vi "OAT Spectral Map (2D array).vi"(0 "scaled signal [EU]":waveform(dbl)={"t0"=timestamp(0 s since 1904-01-01), "dt"=0.0, "Y"=[]}, 1 "dB on? (T)":bool=TRUE, 2 "reset? (F)":bool, 3 "plot type":T9(ring), 5 "speed profile":T8 {"speed [RPM]" format="%.2f"; "time [s]" format="%.2f"}, 7 "pulse/revolution (1)":i32=1, 9 "time/speed segment [s or RPM]":cluster{"start":dbl, "end":dbl, "step size":dbl} {"step size" format="%.2f"; "end" min=0.0 format="%.2f"; "start" min=0.0 format="%.2f"}, 11 "error in (no error)":errorcluster, 12 "max order (auto)":dbl, 13 "windows info":cluster{"window type":u32, "window length":i32}={"window type"=62, "window length"=2048} {"window length" min=2; "window type" items=["None"=0, "Hanning"=1, "Hamming"=2, "Blackman-Harris"=3, "Exact Blackman"=4, "Blackman"=5, "Flat Top"=6, "4 Term B-Harris"=7, "7 Term B-Harris"=8, "Low Sidelobe"=9, "Gaussian"=62]}) -> (4 "spectral map":dbl[][](array[numeric]) format="%.2f", 6 "spectral map info":T7={"scales"={"x scale"={"offset"=0.0, "multiplier"=0.0}, "y scale"={"offset"=0.0, "multiplier"=0.0}}, "unit labels"={"x-axis unit label"="", "y-axis unit label"="", "z-axis unit label"=""}, "plot type"=enum."Frequency-Time", "dB on"=TRUE} {"scales"."y scale"."multiplier" format="%.2f"; "scales"."y scale"."offset" format="%.2f"; "scales"."x scale"."multiplier" format="%.2f"; "scales"."x scale"."offset" format="%.2f"}, 8 "spectrum info":T1={"channel name"="", "description"="", "x-axis units"=0, "spectral info"={"spectrum type"=enum."Power [Magnitude^2]", "linear/dB"=enum."linear", "window"=0, "window size"=0, "FFT size"=0}, "engineering units"=0, "custom label"="", "dB reference [EU]"=0.0, "peak units"=enum."rms", "weighting filter"=0, "spectral density?"=FALSE, "unit label"="", "spectrum skewed?"=FALSE, "complimentary spectrum units"=enum."none"} {"x-axis units" items=["Time (s)"=0, "Frequency-CB (Hz)"=1, "Frequency-CPB (Hz)"=1248, "Frequency-Arbitrary (Hz)"=2357, "Quefrency (s)"=2, "Revolutions (rev)"=3, "Order"=4, "Speed (RPM)"=11, "Speed (rad/s)"=21, "Index"=65535]; "weighting filter" items=["Linear", "A-weighting", "B-weighting", "C-weighting", "ITU-R 468-4", "Dolby", "CCITT", "C-message", "Wb", "Wc", "Wd", "We", "Wf", "Wh", "Wj", "Wk", "Wm", "AES17 20 kHz lowpass", "AES17 40 kHz lowpass", "AES17 20 kHz highpass", "AES17 40 kHz highpass"]; "dB reference [EU]" format="%.2f"; "engineering units" items=["custom..."=0, "V"=1, "A"=21, "C"=30, "pC"=31, "s"=32, "-"=29, "Pa"=2, "N"=20, "g"=3, "m/s^2"=4, "m/s"=5, "m"=6, "mm/s"=12, "mm"=13, "micron/s"=14, "micron"=15, "in/s^2"=7, "in/s"=8, "in"=9, "mil/s"=10, "mil"=11, "rad/s^2"=16, "rad/s"=17, "rad"=18, "deg/s^2"=26, "deg/s"=27, "deg"=28, "RPM"=22, "cycle/s^2"=23, "Hz"=24, "cycle"=25, "strain"=19]; "spectral info"."window" items=["None "=0, "Hanning"=1, "Hamming"=2, "Blackman-Harris"=3, "Exact Blackman"=4, "Blackman"=5, "Flat Top"=6, "4 Term B-Harris "=7, "7 Term B-Harris"=8, "Low Sidelobe"=9, "Force - Exponential"=10, "Gaussian"=62]}, 10 "end reached?":bool, 15 "error out":errorcluster)   [LabVIEW 2017, in "SoundVib_OrderTracking.lvlib"]
doc: "Computes a spectral map of the <B>scaled signal [EU]</B> as a function of time or rotational speed. This VI can return the spectral map as a 2D numeric array, a colormap, or a waterfall graph. Wire data to the <B>scaled signal [EU]</B> input to determine the polymorphic instance to use or manually select the instance."
uses:
  <vilib>/addons/Sound and Vibration/Order Analysis/Resample Order Tracking/SoundVib_OrderTracking.lvlib
  <vilib>/addons/Sound and Vibration/Order Analysis/Tach Process/SubVIs/speed profile.ctl
  <vilib>/addons/Sound and Vibration/Order Analysis/Resample Order Tracking/SubVIs/Spectral Map Info.ctl
  <vilib>/addons/_NISVFA/_Shared subVIs/Controls/svc_Spectrum Info.ctl
  <vilib>/addons/_NISVFA/_Shared subVIs/Controls/svc_X-Axis Units.ctl
  <vilib>/addons/_NISVFA/_Shared subVIs/Controls/svc_Spectrum Type.ctl
  <vilib>/addons/_NISVFA/_Shared subVIs/Controls/svc_Engineering Units Text Ring.ctl
  <vilib>/addons/_NISVFA/_Shared subVIs/Controls/svc_Weighting Filter Text Ring.ctl
  <vilib>/addons/_NISVFA/_Shared subVIs/Controls/svc_Complimentary Spectrum Units.ctl
  <vilib>/addons/_NISVFA/_Shared subVIs/Common/svc_Check for Waveform Parameter Continuity (no state).vi
  <vilib>/addons/Sound and Vibration/Order Analysis/Resample Order Tracking/OAT Convert to Even Angle Signal (1 Channel).vi
  <vilib>/addons/_NISVFA/_Shared subVIs/Common/svc_Engineering Units to Unit Label.vi
  <vilib>/addons/_NISVFA/_Shared subVIs/Common/svc_Unit Label to Engineering Units.vi
  <vilib>/addons/Sound and Vibration/Order Analysis/Resample Order Tracking/SoundVib_Resampling.lvlib
  <vilib>/addons/Sound and Vibration/Order Analysis/Tach Process/SoundVib_TachProcess.lvlib
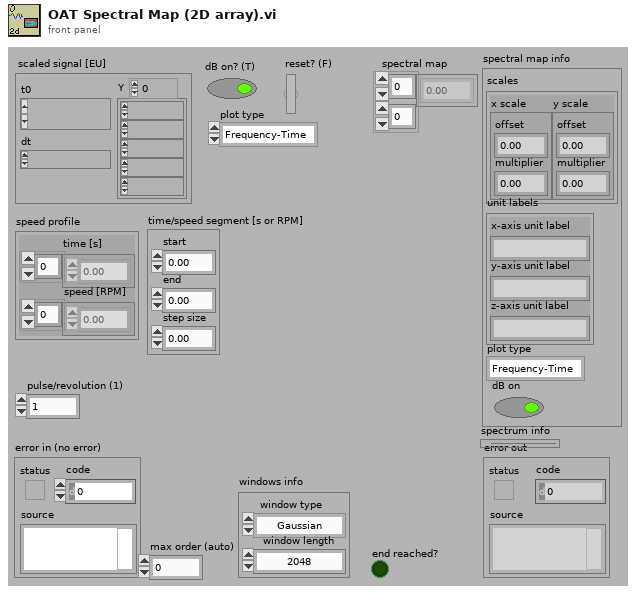
[diagram p1: front panel]
types:
  T1 = typedef "svc_Spectrum Info.ctl" = cluster{"channel name":string, "description":string, "x-axis units":T2, "spectral info":cluster{"spectrum type":T3, "linear/dB":enum16{"linear", "dB"}, "window":u16, "window size":i32, "FFT size":i32}, "engineering units":T4, "custom label":string, "dB reference [EU]":dbl, "peak units":enum16{"rms", "peak", "peak-peak"}, "weighting filter":T5, "spectral density?":bool, "unit label":string, "spectrum skewed?":bool, "complimentary spectrum units":T6}
  T2 = typedef "svc_X-Axis Units.ctl" = u16
  T3 = typedef "svc_Spectrum Type.ctl" = enum16{"FFT Spectrum [complex]", "Amplitude [Magnitude]", "Power [Magnitude^2]", "Cross Spectrum [complex]", "Frequency Response [Complex]"}
  T4 = typedef "svc_Engineering Units Text Ring.ctl" = u16
  T5 = typedef "svc_Weighting Filter Text Ring.ctl" = u16
  T6 = typedef "svc_Complimentary Spectrum Units.ctl" = enum16{"none", "radians", "degrees", "cycles", "imaginary"}
  T7 = typedef "SoundVib_Resampling.lvlib/Spectral Map Info.ctl" = cluster{"scales":cluster{"x scale":cluster{"offset":dbl, "multiplier":dbl}, "y scale":cluster{"offset":dbl, "multiplier":dbl}}, "unit labels":cluster{"x-axis unit label":string, "y-axis unit label":string, "z-axis unit label":string}, "plot type":enum16{"Frequency-Time", "Time-Frequency", "Order-Time", "Time-Order", "Frequency-RPM", "RPM-Frequency", "Order-RPM", "RPM-Order"}, "dB on":bool}
  T8 = typedef "SoundVib_TachProcess.lvlib/speed profile.ctl" = cluster{"time [s]":dbl[], "speed [RPM]":dbl[]}
  T9 = enum16{"Frequency-Time", "Time-Frequency", "Order-Time", "Time-Order", "Frequency-RPM", "RPM-Frequency", "Order-RPM", "RPM-Order"}
  T10 = cluster{"dt":bool, "t0 continuity":bool, "array length":bool, "channel info":bool, "name":bool}
  T11 = cluster{"Z axis unit label":string, "Z axis unit label":string, "Z axis unit label":string}
  T12 = cluster{"X scale":cluster{"offset":dbl, "multiplier":dbl}, "Y scale":cluster{"offset":dbl, "multiplier":dbl}}
  T13 = cluster{"start (s)":dbl, "end (s)":dbl, "step (s)":dbl}
  T14 = typedef "svc_Channel Info.ctl" = cluster{"sensor sensitivity":dbl, "engineering units":T4, "dB reference":dbl, "custom label":string, "weighting filter":T5, "pregain":dbl}
  T15 = cluster{"Y scale":cluster{"offset":dbl, "multiplier":dbl}, "X scale":cluster{"offset":dbl, "multiplier":dbl}}
  T16 = cluster{string, string, "Z axis unit label":string}
  T17 = cluster{"scales":cluster{"X scale":cluster{"offset":dbl, "multiplier":dbl}, "Y scale":cluster{"offset":dbl, "multiplier":dbl}}, cluster{"Z axis unit label":string, "Z axis unit label":string, "Z axis unit label":string}, "plot type":enum16{"Frequency-Time", "Time-Frequency", "Order-Time", "Time-Order", "Frequency-RPM", "RPM-Frequency", "Order-RPM", "RPM-Order"}, "dB on? (T)":bool}
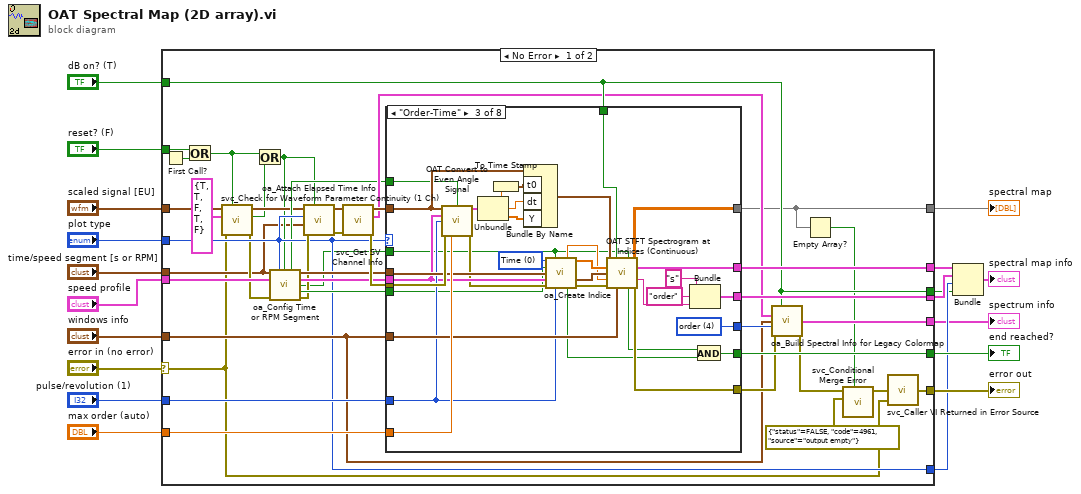
[diagram p0: block diagram]
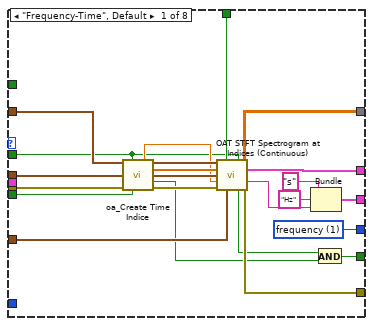
[diagram p2: hidden frame]
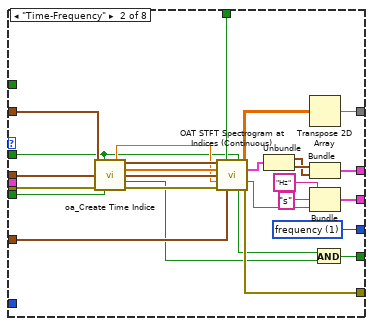
[diagram p3: hidden frame]
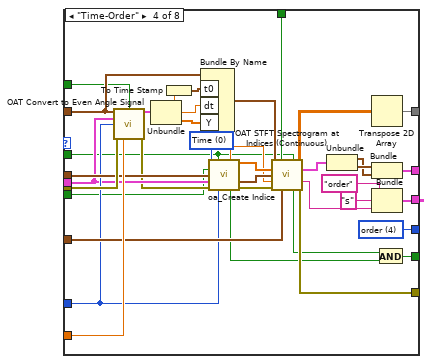
[diagram p4: hidden frame]
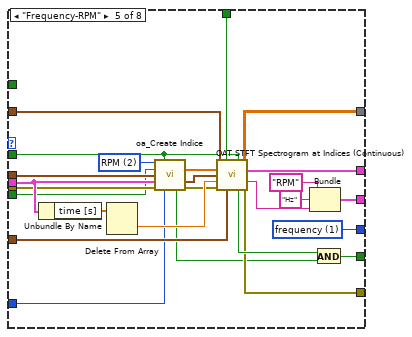
[diagram p5: hidden frame]
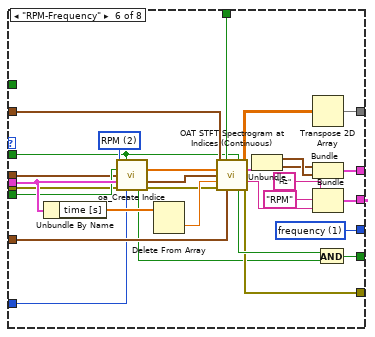
[diagram p6: hidden frame]
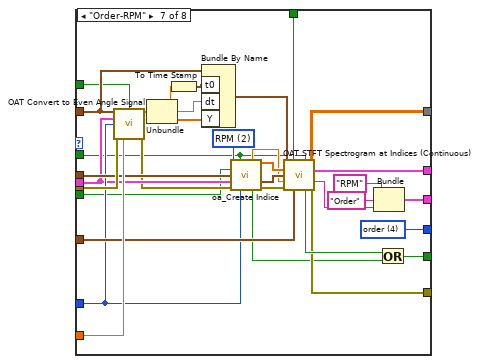
[diagram p7: hidden frame]
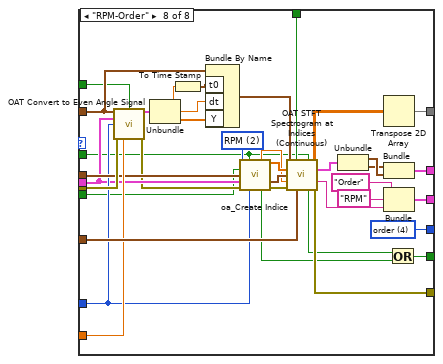
[diagram p8: hidden frame]
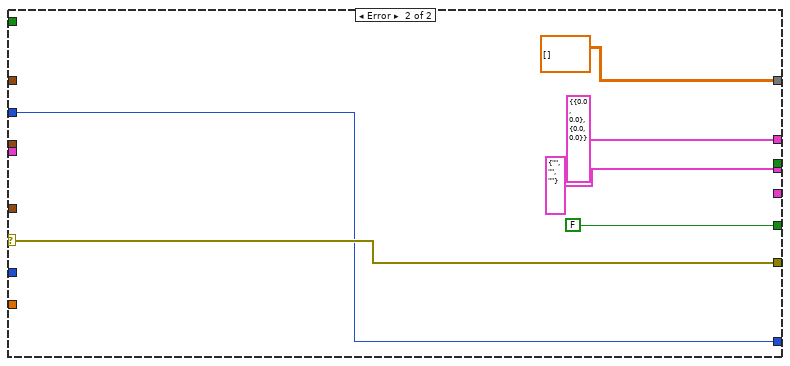
[diagram p9: hidden frame]
diagram:
  n1 = case shown="No Error" "error in (no error)" {
    selector: "error in (no error)" -> [w20 w315]
    tunnel: [w21 w315] -> w18
    tunnel: "time/speed segment [s or RPM]" -> [w28 _]
    tunnel: "plot type" -> [w37 w310]
    tunnel: "windows info" -> [w45 _]
    tunnel: "scaled signal [EU]" -> [w34 _]
    tunnel: "dB on? (T)" -> [w51 _]
    tunnel: [w24 dbl[][] [] ("spectral map")] -> w14
    tunnel: [w59 T12 {"X scale"={"offset"=0.0, "multiplier"=0.0}, "Y scale"={"offset"=0.0, "multiplier"=0.0}} ("scales")] -> w8
    tunnel: [w58 FALSE] -> w13
    tunnel: [w57 T11 {"Z axis unit label"="", "Z axis unit label"="", "Z axis unit label"=""}] -> w7
    tunnel: "speed profile" -> [w43 _]
    tunnel: "pulse/revolution (1)" -> [w56 _]
    tunnel: "max order (auto)" -> [w55 _]
    tunnel: [w37 w310] -> w6
    tunnel: "reset? (F)" -> [w53 _]
    tunnel: [w52 _] -> w2
    tunnel: [w51 _] -> w1
    frame No Error {
      n2 = First Call?() -> (First Call?: T/F=w54:bool)
      n3 = Or(x=w53, y=w54) -> (x .or. y?=w31:bool)
      n4 = call <vilib>:"svc_Check for Waveform Parameter Continuity (1 Ch).vi"("restart averaging (F)"=w31, "error in (no error)"=w20, "checks for channel parameter change"=T10 {"dt"=TRUE, "t0 continuity"=TRUE, "array length"=FALSE, "channel info"=TRUE, "name"=FALSE}, "scaled signal [EU]"=w34) -> ("error out"=w32:errorcluster, "waveform parameter changed"=w30:bool, "dup scaled signal [EU]"=w33:waveform(dbl))  [unwired: 2 in, 3 out]
      n5 = Or(x=w31, y=w30) -> (x .or. y?=w29:bool)
      n6 = call <vilib>:"oa_Config Time or RPM Segment.vi"("time segment"=w28, "plot type"=w37, "reset in"=w29, "speed profile"=w43, "error in (no error)"=w32) -> ("reset resampling"=w35:bool, "time segment out"=w44:T13, "speed profile out"=w42:T8, "reset out"=w36:bool, "step found?"=w41:bool, "error out"=w40:errorcluster)  [unwired: 5 in]
      n7 = call <vilib>:"oa_Attach Elapsed Time Info.vi"("reset? (F)"=w29, "error in (no error)"=w40, "time/speed segment [s or rpm]"=w28, "plot type"=w37, "scaled signal [EU]"=w33) -> ("error out"=w39:errorcluster, "scaled signal [EU] out"=w38:waveform(dbl))  [unwired: 5 in]
      n8 = call <vilib>:"svc_Get SV Channel Info.vi"("error in (no error)"=w39, "scaled signal [EU]"=w38) -> ("error out"=w48:errorcluster, "channel info"=w47:T14, "dup scaled signal [EU]"=w49:waveform(dbl))  [unwired: 4 in, 3 out]
      n9 = case shown="\"Order-Time\"" w37 {
        tunnel: w49 -> [w64 w87 w126 w160 w190 w218 w252 w286]
        tunnel: w44 -> [w69 w91 w123 w157 w189 w214 w248 w282]
        tunnel: w51 -> [w82 w109 w135 w173 w202 w228 w256 w296]
        tunnel: [w81 w96 w132 w161 w201 w229 w262 w295] -> w24
        tunnel: [w80 w97 w131 w162 w200 w226 w261 w294] -> w59
        tunnel: [w79 w107 w133 w171 w197 w223 w257 w292] -> w50
        tunnel: [w77 w105 w114 w151 w198 w224 w258 w287] -> w58
        tunnel: [w73 w103 w127 w168 w199 w225 w260 w293] -> w57
        tunnel: w48 -> [w61 w85 w142 w180 w185 w210 w255 w291]
        tunnel: w42 -> [_ _ w118 w152 w192 w216 w244 w280]
        tunnel: w56 -> [_ _ w119 w153 w184 w212 w245 w281]
        tunnel: w55 -> [_ _ w143 w181 _ _ w254 w289]
        tunnel: w45 -> [w72 w95 w134 w172 w203 w227 w253 w290]
        tunnel: [w71 w94 w125 w159 w196 w222 w251 w285] -> w46
        tunnel: w41 -> [w66 w92 w115 w146 w183 w215 w240 w274]
        tunnel: w36 -> [w60 w83 w111 w145 w182 w208 w239 w273]
        tunnel: w35 -> [_ _ w110 w144 _ _ w238 w272]
        frame "Frequency-Time", Default {
          w71 = u16 1 items=["time"=0, "frequency"=1, "quefrency"=2, "revolutions"=3, "order"=4, "rpm"=11] ("x-axis units")
          n10 = call <vilib>:"oa_Create Time Indice.vi"("scaled signal [EU]"=w64, "reset? (True)"=w60, "steps"=w69, "error in (no error)"=w61, "step found?(F)"=w66) -> ("signal processed"=w62:dbl, "scaled signal [EU] dup"=w63:waveform(dbl), "time indices"=w68:dbl[], "scale"=w67:cluster{"offset":dbl, "multiplier":dbl}, "finished?"=w65:bool, "error out"=w70:errorcluster)  [unwired: 5 in]
          n11 = call <vilib>:"OAT STFT Spectrogram at Indices (Continuous).vi"("resampled signal"=w63, "dB On (T)"=w82, "reset? (True)"=w60, "time indices"=w68, "X scale in"=w67, "last indices"=w62, "error in (no error)"=w70, "spectral settings"=w72) -> ("spectral map"=w81:dbl[][], "scales"=w80:T12, "Z axis unit label"=w76:string, "finished"=w78:bool, "error out"=w79:errorcluster)  [unwired: 3 in]
          n12 = Bundle("Z axis unit label"="s", "Z axis unit label"="Hz", "Z axis unit label"=w76) -> (w73:T11)  [unwired: 1 in]
          n13 = And(x=w78, y=w65) -> (x .and. y?=w77:bool)
        }
        frame "Time-Frequency" {
          w94 = u16 1 items=["time"=0, "frequency"=1, "quefrency"=2, "revolutions"=3, "order"=4, "rpm"=11] ("x-axis units")
          n14 = call <vilib>:"oa_Create Time Indice.vi"("scaled signal [EU]"=w87, "reset? (True)"=w83, "steps"=w91, "error in (no error)"=w85, "step found?(F)"=w92) -> ("signal processed"=w84:dbl, "scaled signal [EU] dup"=w86:waveform(dbl), "time indices"=w90:dbl[], "scale"=w89:cluster{"offset":dbl, "multiplier":dbl}, "finished?"=w88:bool, "error out"=w93:errorcluster)  [unwired: 5 in]
          n15 = call <vilib>:"OAT STFT Spectrogram at Indices (Continuous).vi"("resampled signal"=w86, "dB On (T)"=w109, "reset? (True)"=w83, "time indices"=w90, "X scale in"=w89, "last indices"=w84, "error in (no error)"=w93, "spectral settings"=w95) -> ("spectral map"=w108:dbl[][], "scales"=w100:T12, "Z axis unit label"=w104:string, "finished"=w106:bool, "error out"=w107:errorcluster)  [unwired: 3 in]
          n16 = Unbundle(w100) -> ("X scale"=w98:cluster{"offset":dbl, "multiplier":dbl}, "Y scale"=w99:cluster{"offset":dbl, "multiplier":dbl})
          n17 = Transpose 2D Array(2D array=w108) -> (transposed array=w96:dbl[][])
          n18 = Bundle("Y scale"=w99, "X scale"=w98) -> (w97:T15)  [unwired: 1 in]
          n19 = Bundle("Z axis unit label"="Hz", "Z axis unit label"="s", "Z axis unit label"=w104) -> (w103:T11)  [unwired: 1 in]
          n20 = And(x=w106, y=w88) -> (x .and. y?=w105:bool)
        }
        frame "Order-Time" {
          w124 = u16 0 items=["Time", "Revolution", "RPM"] ("X axis selection")
          w125 = u16 4 items=["time"=0, "frequency"=1, "quefrency"=2, "revolutions"=3, "order"=4, "rpm"=11] ("x-axis units")
          n21 = call-poly <vilib>:"OAT Convert to Even Angle Signal.vi"("scaled signal [EU]"=w126, "reset? (F)"=w110, "speed profile"=w118, "pulse/revolution (1)"=w119, "error in (no error)"=w142, "max order (auto)"=w143) -> ("even-angle signal"=w141:cluster{"r0":dbl, "dr":dbl, "Y":dbl[]}, "error out"=w117:errorcluster)  [unwired: 5 in, 3 out]
          n22 = Unbundle(w141) -> ("r0"=w137:dbl, "dr"=w138:dbl, "Y"=w139:dbl[])
          n23 = To Time Stamp(1:w137) -> (0:w136:timestamp)
          n24 = Bundle By Name(cluster=w126, "t0"=w136, "dt"=w138, "Y"=w139) -> (w140:waveform(dbl))
          n25 = call <vilib>:"oa_Create Indice.vi"("X axis selection"=w124, "reset?(F)"=w111, "step found?(F)"=w115, "steps input"=w123, "speed profile"=w118, "error in (no error)"=w117, "pulse/revolution (1)"=w119) -> ("last rev"=w120:dbl, "rev indice"=w121:dbl[], "scale"=w122:cluster{"offset":dbl, "multiplier":dbl}, "reach end?"=w112:bool, "error out"=w116:errorcluster)  [unwired: 2 in, 2 out]
          n26 = call <vilib>:"OAT STFT Spectrogram at Indices (Continuous).vi"("resampled signal"=w140, "dB On (T)"=w135, "reset? (True)"=w111, "time indices"=w121, "X scale in"=w122, "last indices"=w120, "error in (no error)"=w116, "spectral settings"=w134) -> ("spectral map"=w132:dbl[][], "scales"=w131:T12, "Z axis unit label"=w130:string, "finished"=w113:bool, "error out"=w133:errorcluster)  [unwired: 3 in]
          n27 = Bundle("s", "order", "Z axis unit label"=w130) -> (w127:T16)  [unwired: 1 in]
          n28 = And(x=w113, y=w112) -> (x .and. y?=w114:bool)
        }
        frame "Time-Order" {
          w158 = u16 0 items=["Time", "Revolution", "RPM"] ("X axis selection")
          w159 = u16 4 items=["time"=0, "frequency"=1, "quefrency"=2, "revolutions"=3, "order"=4, "rpm"=11] ("x-axis units")
          n29 = call-poly <vilib>:"OAT Convert to Even Angle Signal.vi"("scaled signal [EU]"=w160, "reset? (F)"=w144, "speed profile"=w152, "pulse/revolution (1)"=w153, "error in (no error)"=w180, "max order (auto)"=w181) -> ("even-angle signal"=w179:cluster{"r0":dbl, "dr":dbl, "Y":dbl[]}, "error out"=w148:errorcluster)  [unwired: 5 in, 3 out]
          n30 = Unbundle(w179) -> ("r0"=w175:dbl, "dr"=w176:dbl, "Y"=w177:dbl[])
          n31 = To Time Stamp(1:w175) -> (0:w174:timestamp)
          n32 = Bundle By Name(cluster=w160, "t0"=w174, "dt"=w176, "Y"=w177) -> (w178:waveform(dbl))
          n33 = call <vilib>:"oa_Create Indice.vi"("X axis selection"=w158, "reset?(F)"=w145, "step found?(F)"=w146, "steps input"=w157, "speed profile"=w152, "error in (no error)"=w148, "pulse/revolution (1)"=w153) -> ("last rev"=w154:dbl, "rev indice"=w155:dbl[], "scale"=w156:cluster{"offset":dbl, "multiplier":dbl}, "reach end?"=w149:bool, "error out"=w147:errorcluster)  [unwired: 2 in, 2 out]
          n34 = call <vilib>:"OAT STFT Spectrogram at Indices (Continuous).vi"("resampled signal"=w178, "dB On (T)"=w173, "reset? (True)"=w145, "time indices"=w155, "X scale in"=w156, "last indices"=w154, "error in (no error)"=w147, "spectral settings"=w172) -> ("spectral map"=w170:dbl[][], "scales"=w165:T12, "Z axis unit label"=w169:string, "finished"=w150:bool, "error out"=w171:errorcluster)  [unwired: 3 in]
          n35 = Unbundle(w165) -> ("X scale"=w163:cluster{"offset":dbl, "multiplier":dbl}, "Y scale"=w164:cluster{"offset":dbl, "multiplier":dbl})
          n36 = Transpose 2D Array(2D array=w170) -> (transposed array=w161:dbl[][])
          n37 = Bundle("Y scale"=w164, "X scale"=w163) -> (w162:T15)  [unwired: 1 in]
          n38 = Bundle("order", "s", "Z axis unit label"=w169) -> (w168:T16)  [unwired: 1 in]
          n39 = And(x=w150, y=w149) -> (x .and. y?=w151:bool)
        }
        frame "Frequency-RPM" {
          w193 = u16 2 items=["Time", "Revolution", "RPM"] ("X axis selection")
          w196 = u16 1 items=["time"=0, "frequency"=1, "quefrency"=2, "revolutions"=3, "order"=4, "rpm"=11] ("x-axis units")
          n40 = Unbundle By Name(w192) -> ("time [s]"=w195:dbl[])
          n41 = Delete From Array(array=w195) -> (deleted portion=w194:dbl)  [unwired: 2 in, 1 out]
          n42 = call <vilib>:"oa_Create Indice.vi"("X axis selection"=w193, "reset?(F)"=w182, "step found?(F)"=w183, "steps input"=w189, "speed profile"=w192, "error in (no error)"=w185, "pulse/revolution (1)"=w184) -> ("time indice"=w191:dbl[], "scale"=w188:cluster{"offset":dbl, "multiplier":dbl}, "reach end?"=w187:bool, "error out"=w186:errorcluster)  [unwired: 2 in, 3 out]
          n43 = call <vilib>:"OAT STFT Spectrogram at Indices (Continuous).vi"("resampled signal"=w190, "dB On (T)"=w202, "reset? (True)"=w182, "time indices"=w191, "X scale in"=w188, "last indices"=w194, "error in (no error)"=w186, "spectral settings"=w203) -> ("spectral map"=w201:dbl[][], "scales"=w200:T12, "Z axis unit label"=w206:string, "finished"=w207:bool, "error out"=w197:errorcluster)  [unwired: 3 in]
          n44 = Bundle("Z axis unit label"="RPM", "Z axis unit label"="Hz", "Z axis unit label"=w206) -> (w199:T11)  [unwired: 1 in]
          n45 = And(x=w207, y=w187) -> (x .and. y?=w198:bool)
        }
        frame "RPM-Frequency" {
          w219 = u16 2 items=["Time", "Revolution", "RPM"] ("X axis selection")
          w222 = u16 1 items=["time"=0, "frequency"=1, "quefrency"=2, "revolutions"=3, "order"=4, "rpm"=11] ("x-axis units")
          n46 = Unbundle By Name(w216) -> ("time [s]"=w221:dbl[])
          n47 = call <vilib>:"oa_Create Indice.vi"("X axis selection"=w219, "reset?(F)"=w208, "step found?(F)"=w215, "steps input"=w214, "speed profile"=w216, "error in (no error)"=w210, "pulse/revolution (1)"=w212) -> ("time indice"=w217:dbl[], "scale"=w213:cluster{"offset":dbl, "multiplier":dbl}, "reach end?"=w211:bool, "error out"=w209:errorcluster)  [unwired: 2 in, 3 out]
          n48 = Delete From Array(array=w221) -> (deleted portion=w220:dbl)  [unwired: 2 in, 1 out]
          n49 = call <vilib>:"OAT STFT Spectrogram at Indices (Continuous).vi"("resampled signal"=w218, "dB On (T)"=w228, "reset? (True)"=w208, "time indices"=w217, "X scale in"=w213, "last indices"=w220, "error in (no error)"=w209, "spectral settings"=w227) -> ("spectral map"=w237:dbl[][], "scales"=w230:T12, "Z axis unit label"=w235:string, "finished"=w236:bool, "error out"=w223:errorcluster)  [unwired: 3 in]
          n50 = Unbundle(w230) -> ("X scale"=w232:cluster{"offset":dbl, "multiplier":dbl}, "Y scale"=w231:cluster{"offset":dbl, "multiplier":dbl})
          n51 = Transpose 2D Array(2D array=w237) -> (transposed array=w229:dbl[][])
          n52 = Bundle("Y scale"=w231, "X scale"=w232) -> (w226:T15)  [unwired: 1 in]
          n53 = Bundle("Z axis unit label"="Hz", "Z axis unit label"="RPM", "Z axis unit label"=w235) -> (w225:T11)  [unwired: 1 in]
          n54 = And(x=w236, y=w211) -> (x .and. y?=w224:bool)
        }
        frame "Order-RPM" {
          w250 = u16 2 items=["Time", "Revolution", "RPM"] ("X axis selection")
          w251 = u16 4 items=["time"=0, "frequency"=1, "quefrency"=2, "revolutions"=3, "order"=4, "rpm"=11] ("x-axis units")
          n55 = call-poly <vilib>:"OAT Convert to Even Angle Signal.vi"("scaled signal [EU]"=w252, "reset? (F)"=w238, "speed profile"=w244, "pulse/revolution (1)"=w245, "error in (no error)"=w255, "max order (auto)"=w254) -> ("even-angle signal"=w271:cluster{"r0":dbl, "dr":dbl, "Y":dbl[]}, "error out"=w242:errorcluster)  [unwired: 5 in, 3 out]
          n56 = Unbundle(w271) -> ("r0"=w268:dbl, "dr"=w269:dbl, "Y"=w270:dbl[])
          n57 = To Time Stamp(1:w268) -> (0:w266:timestamp)
          n58 = Bundle By Name(cluster=w252, "t0"=w266, "dt"=w269, "Y"=w270) -> (w267:waveform(dbl))
          n59 = call <vilib>:"oa_Create Indice.vi"("X axis selection"=w250, "reset?(F)"=w239, "step found?(F)"=w240, "steps input"=w248, "speed profile"=w244, "error in (no error)"=w242, "pulse/revolution (1)"=w245) -> ("last rev"=w243:dbl, "rev indice"=w246:dbl[], "scale"=w247:cluster{"offset":dbl, "multiplier":dbl}, "reach end?"=w249:bool, "error out"=w241:errorcluster)  [unwired: 2 in, 2 out]
          n60 = call <vilib>:"OAT STFT Spectrogram at Indices (Continuous).vi"("resampled signal"=w267, "dB On (T)"=w256, "reset? (True)"=w239, "time indices"=w246, "X scale in"=w247, "last indices"=w243, "error in (no error)"=w241, "spectral settings"=w253) -> ("spectral map"=w262:dbl[][], "scales"=w261:T12, "Z axis unit label"=w265:string, "finished"=w259:bool, "error out"=w257:errorcluster)  [unwired: 3 in]
          n61 = Bundle("RPM", "Order", "Z axis unit label"=w265) -> (w260:T16)  [unwired: 1 in]
          n62 = Or(x=w259, y=w249) -> (x .or. y?=w258:bool)
        }
        frame "RPM-Order" {
          w284 = u16 2 items=["Time", "Revolution", "RPM"] ("X axis selection")
          w285 = u16 4 items=["time"=0, "frequency"=1, "quefrency"=2, "revolutions"=3, "order"=4, "rpm"=11] ("x-axis units")
          n63 = call-poly <vilib>:"OAT Convert to Even Angle Signal.vi"("scaled signal [EU]"=w286, "reset? (F)"=w272, "speed profile"=w280, "pulse/revolution (1)"=w281, "error in (no error)"=w291, "max order (auto)"=w289) -> ("even-angle signal"=w308:cluster{"r0":dbl, "dr":dbl, "Y":dbl[]}, "error out"=w276:errorcluster)  [unwired: 5 in, 3 out]
          n64 = Unbundle(w308) -> ("r0"=w305:dbl, "dr"=w306:dbl, "Y"=w307:dbl[])
          n65 = To Time Stamp(1:w305) -> (0:w303:timestamp)
          n66 = Bundle By Name(cluster=w286, "t0"=w303, "dt"=w306, "Y"=w307) -> (w304:waveform(dbl))
          n67 = call <vilib>:"oa_Create Indice.vi"("X axis selection"=w284, "reset?(F)"=w273, "step found?(F)"=w274, "steps input"=w282, "speed profile"=w280, "error in (no error)"=w276, "pulse/revolution (1)"=w281) -> ("last rev"=w277:dbl, "rev indice"=w278:dbl[], "scale"=w279:cluster{"offset":dbl, "multiplier":dbl}, "reach end?"=w283:bool, "error out"=w275:errorcluster)  [unwired: 2 in, 2 out]
          n68 = call <vilib>:"OAT STFT Spectrogram at Indices (Continuous).vi"("resampled signal"=w304, "dB On (T)"=w296, "reset? (True)"=w273, "time indices"=w278, "X scale in"=w279, "last indices"=w277, "error in (no error)"=w275, "spectral settings"=w290) -> ("spectral map"=w309:dbl[][], "scales"=w299:T12, "Z axis unit label"=w302:string, "finished"=w288:bool, "error out"=w292:errorcluster)  [unwired: 3 in]
          n69 = Unbundle(w299) -> ("X scale"=w298:cluster{"offset":dbl, "multiplier":dbl}, "Y scale"=w297:cluster{"offset":dbl, "multiplier":dbl})
          n70 = Transpose 2D Array(2D array=w309) -> (transposed array=w295:dbl[][])
          n71 = Bundle("Y scale"=w297, "X scale"=w298) -> (w294:T15)  [unwired: 1 in]
          n72 = Bundle("Order", "RPM", "Z axis unit label"=w302) -> (w293:T16)  [unwired: 1 in]
          n73 = Or(x=w288, y=w283) -> (x .or. y?=w287:bool)
        }
      }
      n74 = call <vilib>:"oa_Build Spectral Info for Legacy Colormap.vi"("dB on (T)"=w51, "channel info"=w47, "windows info"=w45, "x-axis units"=w46, "error in"=w50) -> ("spectrum info"=w52:T1, "error out"=w25:errorcluster)  [unwired: 9 in]
      n75 = Empty Array?(array=w24) -> (empty?=w23:bool)
      n76 = call <vilib>:"svc_Conditional Merge Error.vi"("merge"=w23, "new error"=errorcluster {"status"=FALSE, "code"=4961, "source"="output empty"}, "error in (no error)"=w25) -> ("error out"=w22:errorcluster)  [unwired: 8 in]
      n77 = call <vilib>:"svc_Caller VI Returned in Error Source.vi"("warning input to caller"=w20, "error in (no error)"=w22) -> ("error out"=w21:errorcluster)  [unwired: 3 in]
    }
    frame Error {
    }
  }
  "spectral map" <- w14
  "end reached?" <- w13
  "error out" <- w18
  "spectrum info" <- w2
  n78 = Bundle("scales"=w8, w7, "plot type"=w6, "dB on? (T)"=w1) -> (→"spectral map info":T17)  [unwired: 1 in]
